vi "AlwaysPID.vi"() -> ()   [LabVIEW 2012]
uses:
  State_Machine_Enum.ctl
  Robot Global Data.vi
  <vilib>/addons/control/pid/NI_PID_pid.lvlib
  <vilib>/addons/control/pid/pid.llb/PID (DBL).vi
panel:
  in  "RightSide":dbl
  in  "LeftSide":dbl
  out "Speed Chart L":dbl(graph)
  out "Speed Chart R":dbl(graph)
  out "Waveform Chart R":dbl(graph)
  in  "MaxRPM":dbl=50.0
  out "Loop Difference":u32
  out "State":T1
  out "Waveform Chart L":dbl(graph)
  in  "Output Range":cluster{"Output Max":dbl, "Output Min":dbl}={"Output Max"=1.0, "Output Min"=0.0} {"Output Min" step=0.1; "Output Max" step=0.1}
  in  "PID Gains":T2={"Proportional Gain (Kc)"=0.015, "Integral Time (Ki, sec)"=0.001, "Derivative Time (Kd, sec)"=0.0} {"Derivative Time (Kd, sec)" min=-0.01 max=1.01 step=0.01; "Integral Time (Ki, sec)" min=-0.01 max=10.0 step=0.001; "Proportional Gain (Kc)" min=-0.1 max=5.1 step=0.001}
  # "Defaults: \nKc: 2.4\nKi:  4.8\nKd: 0.3"
  # "Defaults: \nMax 0\nMin -1"
  # "HOW TO CALCULATE PID VALUES:\n1) Find time to accelerate to max speed. (In this case, \n     .5 sec.) This is T.\n2) Assume delay between start / max acceleration \n     is 1/2 of value in step 1. This is L.\n3) Calculate PID values:\n     P: 1.2 (T/L)\n     I: .6(T/L^2)\n     D: .6T\n(This is the dumbed-down version.)"
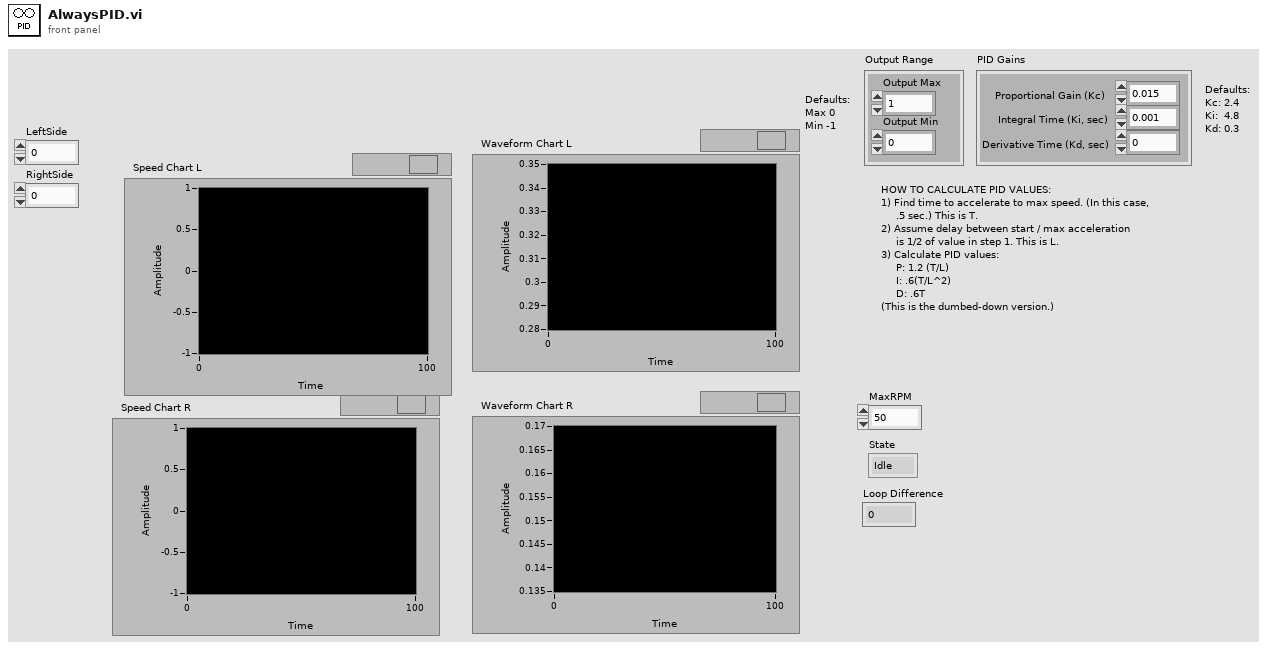
[diagram p1: front panel]
types:
  T1 = typedef "State_Machine_Enum.ctl" = enum16{"Idle", "Start", "Do", "Stop", "Init"}
  T2 = cluster{"Proportional Gain (Kc)":dbl, "Integral Time (Ki, sec)":dbl, "Derivative Time (Kd, sec)":dbl}
  T3 = typedef "WPI_RobotDriveDevRef.ctl" = cluster{"DevStatus":errorcluster, "Motors[]":T4[], "Square Inputs":bool, "Max Output":dbl, "Isochronous":bool}
  T4 = typedef "WPI_MotorControlDeviceRef.ctl" = cluster{"DeviceStatus":errorcluster, "Type":enum16{"PWM", "CAN"}, "PWM":cluster{"Digital Module":T5, "PWM Channel":T6, "DeadBand":T7}, "CAN":cluster{"Device Number":u8, "Control Mode":T8, "Semaphore":T9, "Max Vout":dbl}, "Invert":bool, "TransformRef":T10, "InvTransformRef":T10}
  T5 = typedef "FPGA_TypedefDigitalModule.ctl" = enum16{"Digital Module 1", "Digital Module 2"}
  T6 = typedef "FPGA_DIOPWMChannel.ctl" = enum8{"PWM 1", "PWM 2", "PWM 3", "PWM 4", "PWM 5", "PWM 6", "PWM 7", "PWM 8", "PWM 9", "PWM 10", "Invalid"}
  T7 = typedef "WPI_PWMDeadband.ctl" = cluster{"Name":string, "maxPositivePwm":i32, "minPositivePwm":i32, "centerPwm":i32, "maxNegativePwm":i32, "minNegativePwm":i32, "angularRange":u16}
  T8 = typedef "WPI_CANJaguar_ControlMode.ctl" = enum8{"Percent VBus", "Current", "Speed", "Position", "Voltage"}
  T9 = typedef "Semaphore RefNum" = refnum<k1>
  T10 = typedef "WPI_PWMTransform_ConPane.ctl" = refnum<vi>
  T11 = typedef "LoopDisable.ctl" = cluster{"Climb.vi":bool, "LauncherAngle.vi":bool, "Launcher.vi":bool, "ArmControl.vi":bool, "WinchMotor.vi":bool, "ReadDriveEncoder.vi":bool}
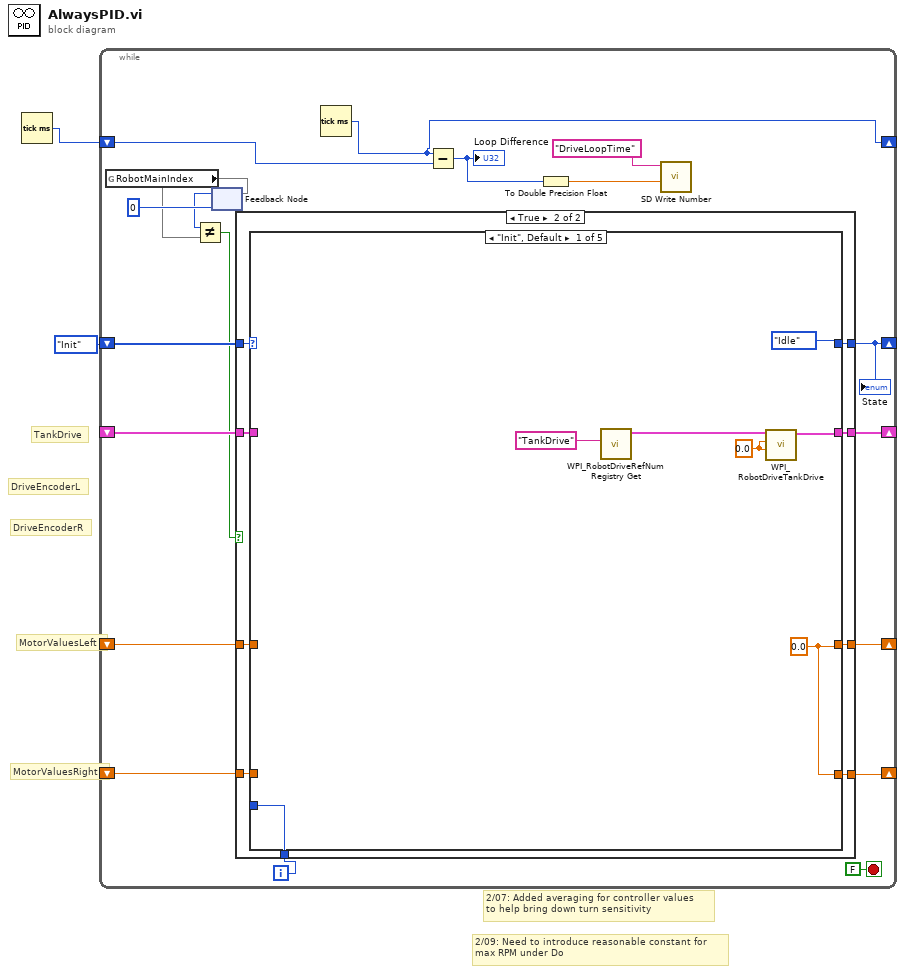
[diagram p0: block diagram]
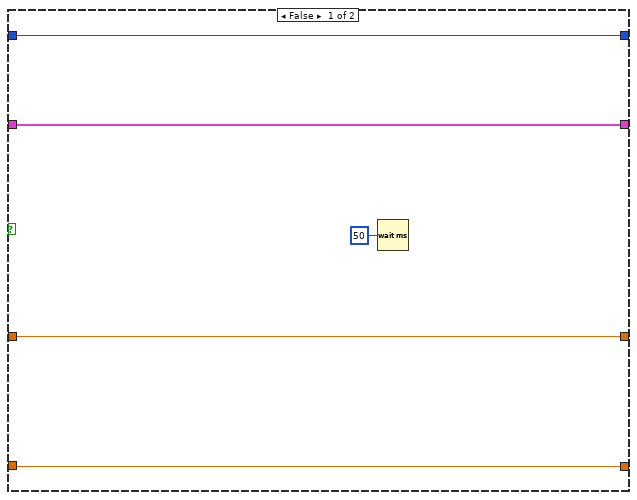
[diagram p2: hidden frame]
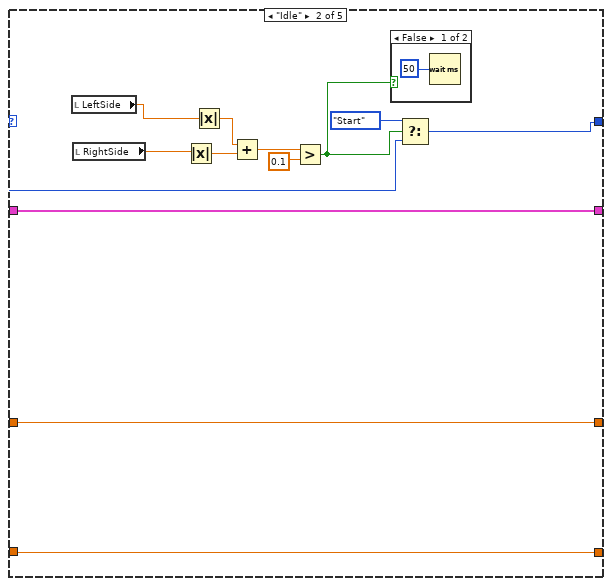
[diagram p3: hidden frame]
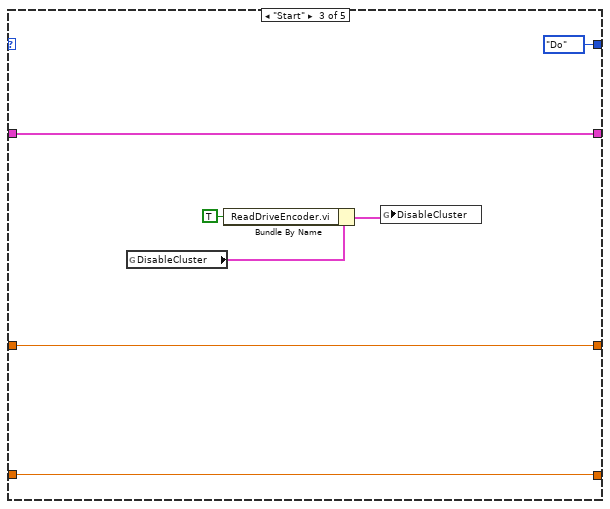
[diagram p5: hidden frame]
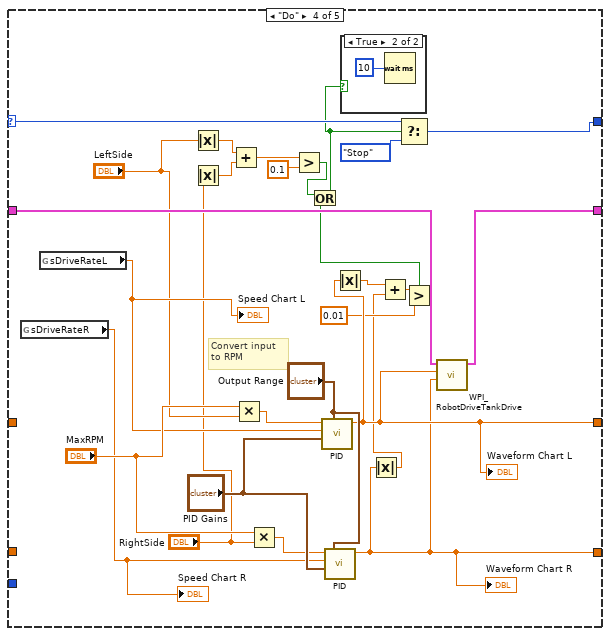
[diagram p6: hidden frame]
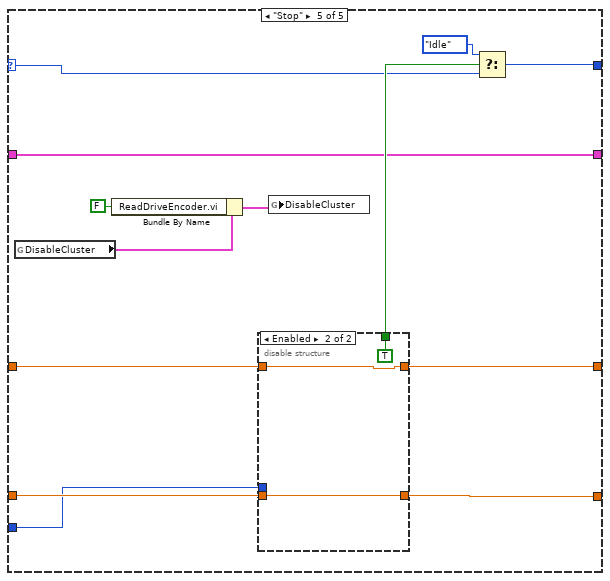
[diagram p8: hidden frame]
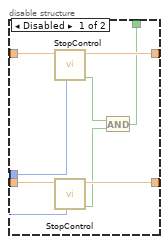
[diagram p9: hidden frame]
diagram:
  # "MotorValuesRight"
  # "MotorValuesLeft"
  # "2/09: Need to introduce reasonable constant for\nmax RPM under Do"
  # "TankDrive"
  # "DriveEncoderR"
  # "DriveEncoderL"
  # "2/07: Added averaging for controller values\nto help bring down turn sensitivity"
  n1 = Tick Count (ms)() -> (millisecond timer value=w1:u32)
  n2 = while {
    shift-right: [w19] -> _
    shift-left: State_Machine_Enum."Init" ("State") -> [w20]
    shift-right: [w18] -> _
    shift-left: _ -> [w17]
    shift-right: [w15] -> _
    shift-left: _ -> [w13]
    shift-right: [w16] -> _
    shift-left: _ -> [w14]
    shift-right: [w7] -> _
    shift-left: w1 -> [w8]
    i -> [w12]
    stop <- FALSE stop-if-true
    n3 = global read "Robot Global Data.vi" "RobotMainIndex"() -> (w4)
    n4 = feedback #1(0 ("TeleopIndex")) -> (w5:i32)
    n5 = Not Equal?(x=w5, y=w4) -> (x != y?=w3:bool)
    n6 = feedback-in #1(w4) -> ()
    n7 = case shown="True" w3 {
      tunnel: w20 -> [w26 w35]
      tunnel: [w26 w34] -> w19
      tunnel: [w25 w33] -> w18
      tunnel: w17 -> [w25 w32]
      tunnel: [w24 w31] -> w16
      tunnel: [w23 w30] -> w15
      tunnel: w14 -> [w24 w29]
      tunnel: w13 -> [w23 w28]
      tunnel: w12 -> [_ w27]
      frame False {
        n8 = Wait (ms)(milliseconds to wait=u32 50) -> ()  [unwired: 1 out]
      }
      frame True {
        n9 = case shown="\"Init\", Default" w35 {
          selector: w35 -> [_ w49 _ w85 w97]
          tunnel: [State_Machine_Enum."Idle" ("State") w48 State_Machine_Enum."Do" ("State") w84 w96] -> w34
          tunnel: [w37 w46 w62 w79 w91] -> w33
          tunnel: w32 -> [_ w46 w62 w80 w91]
          tunnel: [w36 w45 w60 w74 w102] -> w31
          tunnel: [w36 w44 w59 w67 w101] -> w30
          tunnel: w29 -> [_ w45 w60 _ w103]
          tunnel: w28 -> [_ w44 w59 _ w100]
          tunnel: w27 -> [_ _ _ _ w95]
          frame "Init", Default {
            w36 = 0.0
            w39 = 0.0 ("Left axis value")
            n10 = call <vilib>:"WPI_RobotDriveRefNum Registry Get.vi"("refnum name"="TankDrive") -> ("RobotDriveDevRef"=w38:T3)  [unwired: 9 in, 1 out]
            n11 = call <vilib>:"WPI_RobotDriveTankDrive.vi"("Right axis value"=w39, "Left axis value"=w39, "RobotDriveDevRef"=w38) -> ("RobotDriveDevRef"=w37:T3)  [unwired: 6 in, 2 out]
          }
          frame "Idle" {
            n12 = local read "LeftSide"() -> (w42:dbl)
            n13 = local read "RightSide"() -> (w43:dbl)
            n14 = Absolute Value(x=w43) -> (abs(x)=w53:dbl)
            n15 = Absolute Value(x=w42) -> (abs(x)=w54:dbl)
            n16 = Add(x=w54, y=w53) -> (x+y=w52:dbl)
            n17 = Greater?(x=w52, y=0.1) -> (0:w50:bool)
            n18 = case shown="False" w50 {
              frame False {
                n19 = Wait (ms)(milliseconds to wait=u32 50) -> ()  [unwired: 1 out]
              }
              frame True {
              }
            }
            n20 = Select(t=State_Machine_Enum."Start" ("State"), s=w50, f=w49) -> (s? t:f=w48:T1)
          }
          frame "Start" {
            n21 = global read "Robot Global Data.vi" "DisableCluster"() -> (w56:T11)
            n22 = Bundle By Name(cluster=w56, "ReadDriveEncoder.vi"=TRUE) -> (w57:T11)
            n23 = global write "Robot Global Data.vi" "DisableCluster"(w57) -> ()
          }
          frame "Do" {
            # "Convert input \nto RPM"
            n24 = global read "Robot Global Data.vi" "sDriveRateR"() -> (w66:dbl)
            "Speed Chart R" <- w66
            n25 = global read "Robot Global Data.vi" "sDriveRateL"() -> (w65:dbl)
            "Speed Chart L" <- w65
            n26 = Absolute Value(x="LeftSide") -> (abs(x)=w89:dbl)
            n27 = Absolute Value(x="RightSide") -> (abs(x)=w88:dbl)
            n28 = Add(x=w89, y=w88) -> (x+y=w86:dbl)
            n29 = Multiply(x="MaxRPM", y="LeftSide") -> (x*y=w77:dbl)
            n30 = Multiply(x="MaxRPM", y="RightSide") -> (x*y=w78:dbl)
            n31 = Greater?(x=w86, y=0.1) -> (0:w75:bool)
            n32 = call-poly <vilib>:"PID.vi"("output range"="Output Range", "PID gains"="PID Gains", "process variable"=w65, "setpoint"=w77) -> ("output"=w74:dbl)  [unwired: 6 in, 1 out]
            "Waveform Chart L" <- w74
            n33 = call-poly <vilib>:"PID.vi"("output range"="Output Range", "PID gains"="PID Gains", "process variable"=w66, "setpoint"=w78) -> ("output"=w67:dbl)  [unwired: 6 in, 1 out]
            "Waveform Chart R" <- w67
            n34 = Absolute Value(x=w74) -> (abs(x)=w71:dbl)
            n35 = Absolute Value(x=w67) -> (abs(x)=w70:dbl)
            n36 = Add(x=w71, y=w70) -> (x+y=w69:dbl)
            n37 = Greater?(x=w69, y=0.01) -> (0:w72:bool)
            n38 = Or(x=w75, y=w72) -> (x .or. y?=w76:bool)
            n39 = case shown="True" w76 {
              frame False {
              }
              frame True {
                n40 = Wait (ms)(milliseconds to wait=u32 10) -> ()  [unwired: 1 out]
              }
            }
            n41 = Select(t=w85, s=w76, f=State_Machine_Enum."Stop" ("State")) -> (s? t:f=w84:T1)
            n42 = call <vilib>:"WPI_RobotDriveTankDrive.vi"("Right axis value"=w67, "Left axis value"=w74, "RobotDriveDevRef"=w80) -> ("RobotDriveDevRef"=w79:T3)  [unwired: 6 in, 2 out]
          }
          frame "Stop" {
            n43 = global read "Robot Global Data.vi" "DisableCluster"() -> (w92:T11)
            n44 = Bundle By Name(cluster=w92, "ReadDriveEncoder.vi"=FALSE) -> (w93:T11)
            n45 = disable-structure shown="Enabled" {
              disable-tunnel: w103 -> [w111 w113]
              disable-tunnel: [w110 w113] -> w102
              disable-tunnel: [w109 w112] -> w101
              disable-tunnel: w100 -> [w108 w112]
              disable-tunnel: [w105 TRUE] -> w99
              disable-tunnel: w95 -> [w104 _]
              frame Disabled {
                n46 = call "StopControl.vi"("Loop Iteration"=w104, "Motor Value"=w111) -> ("Done Stopping"=w107:bool, "New Motor Value"=w110:dbl)  [unwired: 8 in]
                n47 = call "StopControl.vi"("Loop Iteration"=w104, "Motor Value"=w108) -> ("Done Stopping"=w106:bool, "New Motor Value"=w109:dbl)  [unwired: 8 in]
                n48 = And(x=w107, y=w106) -> (x .and. y?=w105:bool)
              }
              frame Enabled {
              }
            }
            n49 = global write "Robot Global Data.vi" "DisableCluster"(w93) -> ()
            n50 = Select(t=State_Machine_Enum."Idle" ("State"), s=w99, f=w97) -> (s? t:f=w96:T1)
          }
        }
      }
    }
    "State" <- w19
    n51 = Tick Count (ms)() -> (millisecond timer value=w7:u32)
    n52 = Subtract(x=w7, y=w8) -> (x-y=w11:u32)
    "Loop Difference" <- w11
    n53 = To Double Precision Float(number=w11) -> (double precision float=w10:dbl)
    n54 = call <vilib>:"SD Write Number.vi"("Numeric"=w10, "Name"="DriveLoopTime") -> ()  [unwired: 8 in, 2 out]
  }
